vi "calcula brewster.vi"(6 "Ángulo Final":dbl, 9 "Ángulo Inicial":dbl, 10 "EJE Y":dbl[](array[numeric]), 11 "EJE X":dbl[](array[numeric])) -> (1 "Ángulo de Brewster":dbl, 2 "Curva FILTRADA":cluster{dbl[], dbl[]}(graph), 3 "Curva de reflectancia":cluster{dbl[], dbl[]}(graph), 4 "Índice de Refracción":dbl, 5 "Numeric Control":dbl)   [LabVIEW 2025, in "Control de MaP.lvlib"]
uses:
  Control de MaP.lvlib
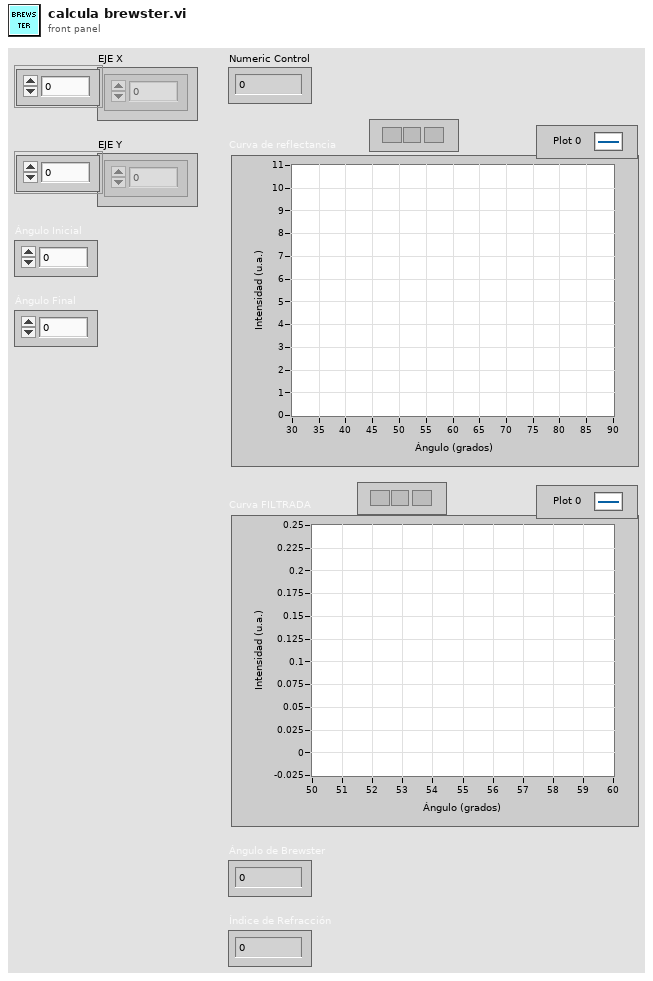
[diagram p1: front panel]
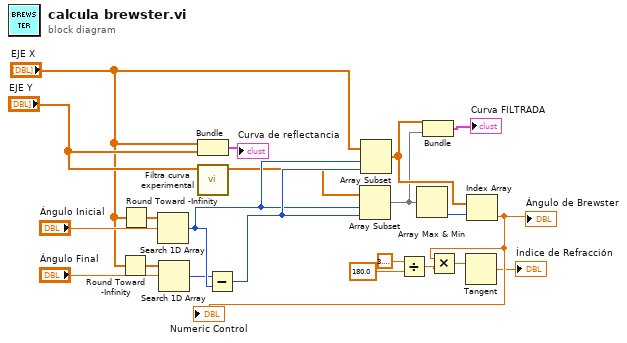
[diagram p0: block diagram]
diagram:
  n1 = Round Toward -Infinity(1:"EJE X") -> (0:w3:dbl[])
  n2 = Round Toward -Infinity(1:"EJE X") -> (0:w1:dbl[])
  n3 = Search 1D Array(1D array=w1, element="Ángulo Inicial") -> (index of element=w11:i32)  [unwired: 1 in]
  n4 = Search 1D Array(1D array=w3, element="Ángulo Final") -> (index of element=w10:i32)  [unwired: 1 in]
  n5 = Bundle("EJE X"="EJE X", "EJE Y"="EJE Y") -> (→"Curva de reflectancia":cluster{"EJE X":dbl[], "EJE Y":dbl[]})  [unwired: 1 in]
  n6 = call "Filtra curva experimental.vi"("Y"="EJE Y") -> ("Y Filtrada"=w6:dbl[])  [unwired: 8 in, 2 out]
  n7 = Subtract(x=w10, y=w11) -> (x-y=w12:i32)
  n8 = Array Subset(array=w6, index=w11, length=w12) -> (w4:dbl[])
  n9 = Array Subset(array="EJE X", index=w11, length=w12) -> (w5:dbl[])
  n10 = Divide(x=3.141592653589793, y=180.0) -> (x/y=w18:dbl)
  n11 = Array Max & Min(array=w4) -> (min index (indices)=w14:i32)  [unwired: 3 out]
  n12 = Bundle(w5, w4) -> (→"Curva FILTRADA":cluster{dbl[], dbl[]})  [unwired: 1 in]
  n13 = Index Array(array=w5, index=w14) -> (element=w21:dbl)
  "Ángulo de Brewster" <- w21
  "Numeric Control" <- w21
  n14 = Multiply(x=w21, y=w18) -> (x*y=w19:dbl)
  n15 = Tangent(1:w19) -> (0:→"Índice de Refracción":dbl)
